vi "Constuct.vi"(8 "error in (no error)":errorcluster, 11 "CDependencyQueue in":refnum<class "CDependencyQueue.lvclass">) -> (0 "error out":errorcluster, 3 "CDependencyQueue out":refnum<class "CDependencyQueue.lvclass">)   [LabVIEW 2020, in "DependencyInspection.lvlib" / "CDependencyQueue.lvclass"]
uses:
  CDependencyQueue.lvclass
  DependencyQueue.ctl
  CDependencyQueue.lvclass/CDependencyQueue.ctl
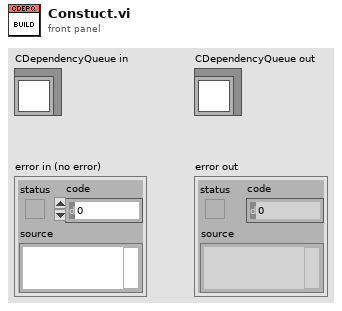
[diagram p1: front panel]
types:
  T1 = typedef "DependencyInspection.lvlib/CDependencyQueue.lvclass/DependencyQueue.ctl" = cluster{"New dependency":path, "Shallow dep?":bool}
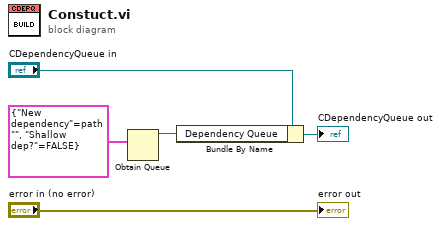
[diagram p0: block diagram]
diagram:
  n1 = Obtain Queue(element data type=T1 {"New dependency"=path "", "Shallow dep?"=FALSE} ("Dep info")) -> (queue out=w1:refnum<queue>)  [unwired: 4 in, 2 out]
  n2 = Bundle By Name(cluster="CDependencyQueue in", "Dependency Queue"=w1) -> (→"CDependencyQueue out":refnum<class "CDependencyQueue.lvclass">)
  "error out" <- "error in (no error)"
